vi "SDcullStatsTable.vi"(7 "SDcut":dbl, 10 "ResultsTable":dbl[][](array[numeric])) -> (0 "InBand":bool[][](array[boolean]), 1 "StatsOut":dbl[][](array[numeric]), 4 "StatsNames":string[](array[string]))   [LabVIEW 2018]
uses:
  <vilib>/Analysis/baseanly.llb/Unimode.vi
  <vilib>/Analysis/NI_AALBase.lvlib
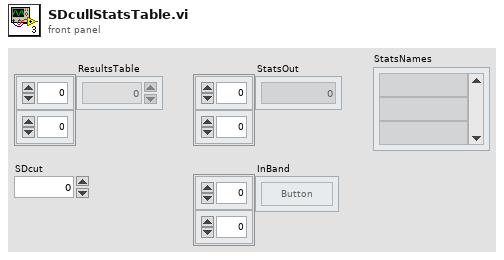
[diagram p1: front panel]
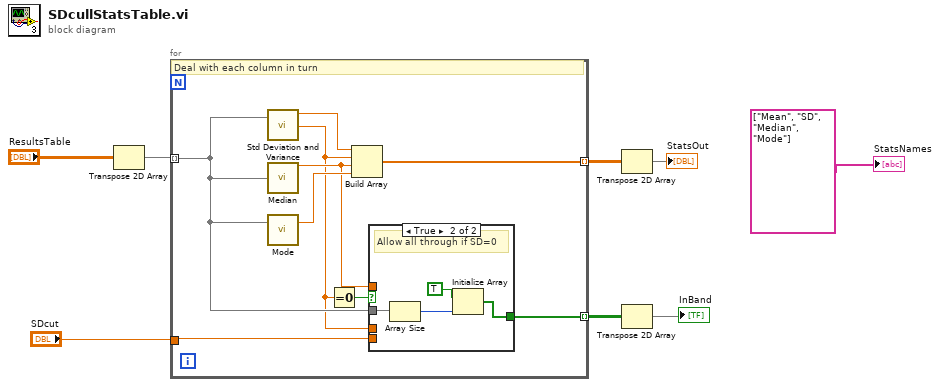
[diagram p0: block diagram]
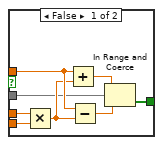
[diagram p2: hidden frame]
diagram:
  n1 = Transpose 2D Array(2D array="ResultsTable") -> (transposed array=w4:dbl[][])
  n2 = for {
    tunnel: w4 -> [w13] mode=indexing
    tunnel: [w16] -> w2 mode=indexing
    tunnel: [w12] -> w5 mode=indexing
    tunnel: "SDcut" -> [w11]
    # "Deal with each column in turn"
    n3 = call <vilib>:"Std Deviation and Variance.vi"("X"=w13) -> ("mean"=w17:dbl, "standard deviation"=w9:dbl)  [unwired: 1 in, 1 out]
    n4 = call <vilib>:"Median.vi"("X"=w13) -> ("median"=w14:dbl)  [unwired: 1 out]
    n5 = call-poly <vilib>:"Mode.vi"("X"=w13) -> ("mode"=w15:dbl)  [unwired: 1 in, 1 out]
    n6 = Equal To 0?(x=w9) -> (x = 0?=w10:bool)
    n7 = Build Array(w17, w9, w14, w15) -> (w16:dbl[])
    n8 = case shown="True" w10 {
      tunnel: w14 -> [w23 _]
      tunnel: w9 -> [w22 _]
      tunnel: w13 -> [w20 w29]
      tunnel: [w19 w28] -> w12
      tunnel: w11 -> [w18 _]
      frame False {
        n9 = Multiply(x=w22, y=w18) -> (x*y=w21:dbl)
        n10 = Add(x=w23, y=w21) -> (x+y=w25:dbl)
        n11 = Subtract(x=w23, y=w21) -> (x-y=w24:dbl)
        n12 = In Range and Coerce(upper limit=w25, x=w20, lower limit=w24) -> (In Range?=w19:bool[])  [unwired: 1 out]
      }
      frame True {
        # "Allow all through if SD=0"
        n13 = Array Size(array=w29) -> (size(s)=w27:i32)
        n14 = Initialize Array(TRUE, w27) -> (w28:bool[])
      }
    }
  }
  n15 = Transpose 2D Array(2D array=w2) -> (transposed array=→"StatsOut":dbl[][])
  n16 = Transpose 2D Array(2D array=w5) -> (transposed array=→"InBand":bool[][])
  "StatsNames" <- string[] ["Mean", "SD", "Median", "Mode"] ("Titles")
